vi "Catch_screw.vi"(7 "櫃子在哪?":enum16{"前面", "左邊", "右邊"}(ring), 8 "Error In":errorcluster) -> (0 "Error Out":errorcluster)   [LabVIEW 2019]
uses:
  WSCbot_V3_Toolkit.lvlibp/WSCBOTV3_Toolkit/IO/LowLevel/PulseCounter.ctl
  WSCbot_V3_Toolkit.lvlibp
panel:
  in  "螺桿高度":dbl(ring)=78.0 items=["物料櫃第一格"=0.0, "物料櫃第二格"=78.0, "螺帽夾取高度"=128.0, "螺帽瞄準"=250.0, "最高"=288.0]
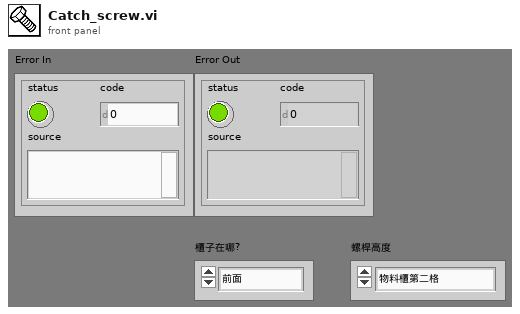
[diagram p1: front panel]
types:
  T1 = enum16{"Right_up", "Right_down", "Left_down", "Left_up", "left", "right", "up", "down"}
  T2 = typedef "WSCbot_V3_Toolkit.lvlibp/PulseCounter.ctl" = enum16{"CH1", "CH2", "CH3", "CH4", "CH5"}
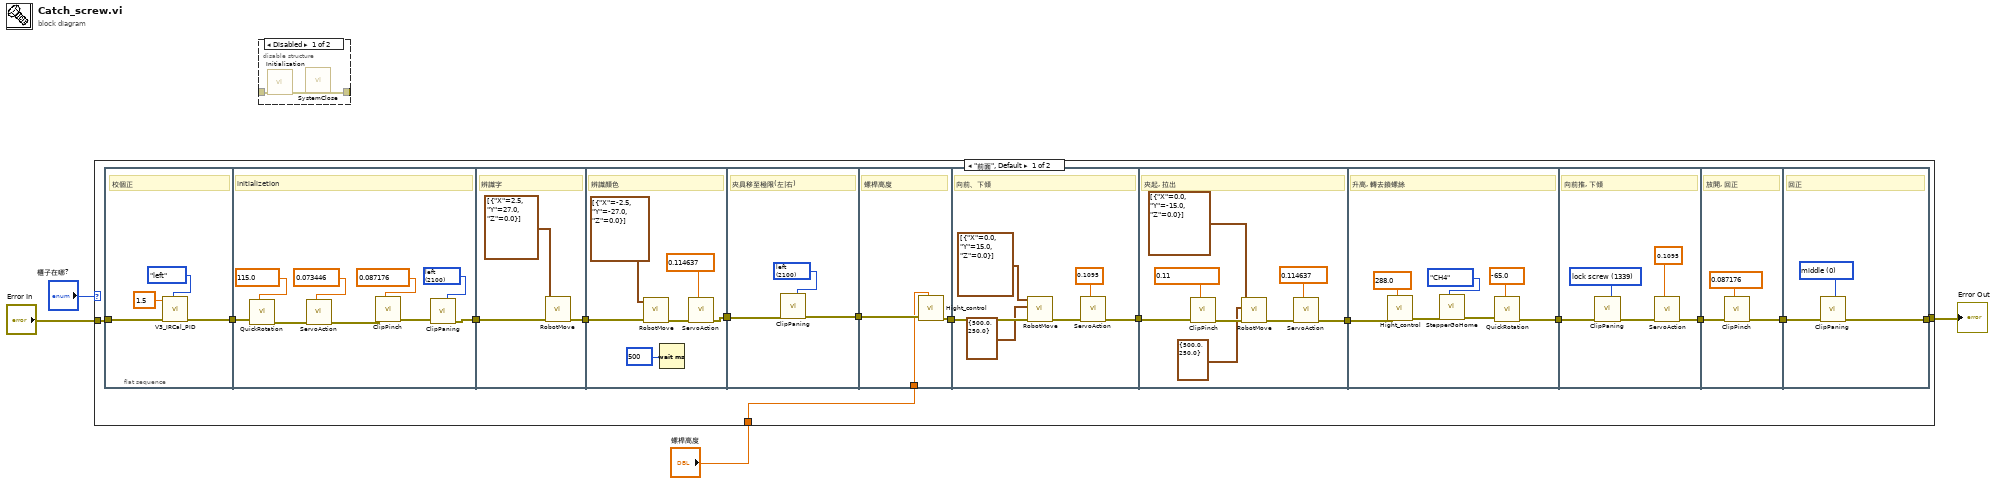
[diagram p0: block diagram]
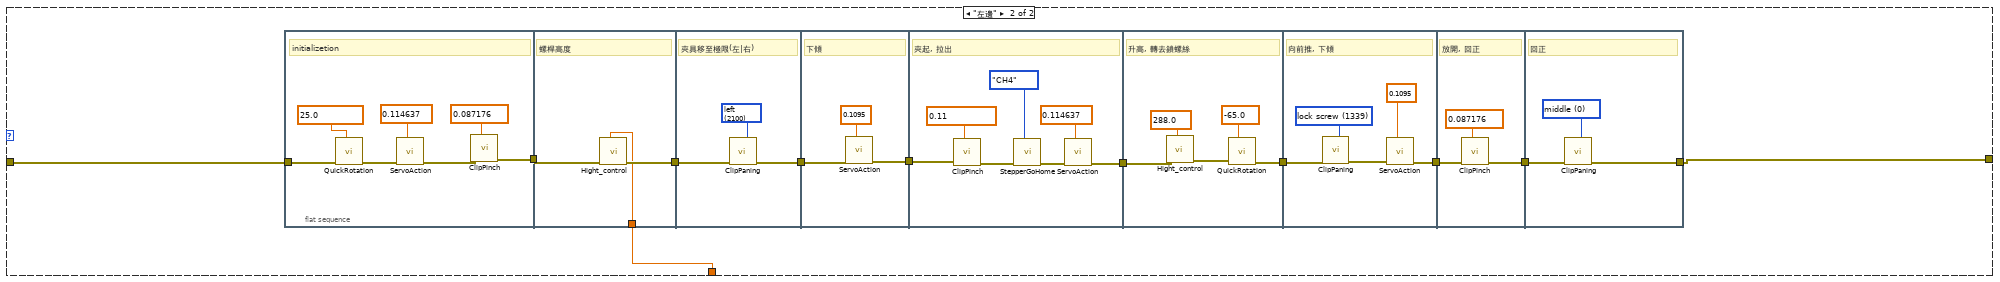
[diagram p2: hidden frame]
diagram:
  n1 = case shown="\"前面\", Default" "櫃子在哪?" {
    tunnel: [w10 w81] -> w4
    tunnel: "Error In" -> [w11 w80]
    tunnel: "螺桿高度" -> [w8 w79]
    frame "前面", Default {
      n2 = flat-sequence {
        tunnel: w11 -> [w21]
        tunnel: [w20] -> w5
        tunnel: [w24] -> w6
        tunnel: w5 -> [w26]
        tunnel: [w34] -> w7
        tunnel: w6 -> [w32]
        tunnel: [w37] -> w18
        tunnel: w7 -> [w40]
        tunnel: w18 -> [w42]
        tunnel: [w41] -> w9
        tunnel: [w45] -> w17
        tunnel: w9 -> [w46]
        tunnel: w8 -> [w44]
        tunnel: w17 -> [w50]
        tunnel: [w52] -> w16
        tunnel: [w58] -> w15
        tunnel: w16 -> [w59]
        tunnel: w15 -> [w65]
        tunnel: [w66] -> w14
        tunnel: w14 -> [w72]
        tunnel: [w68] -> w13
        tunnel: w13 -> [w75]
        tunnel: [w73] -> w12
        tunnel: w12 -> [w77]
        tunnel: [w76] -> w10
        frame #0 {
          # "校個正"
          n3 = call "V3_IRCal_PID.vi"("Direction"=T1."left", "Error In"=w21, "X_distance(V)"=1.5) -> ("Error Out"=w20:errorcluster)  [unwired: 7 in, 1 out]
        }
        frame #1 {
          w23 = 2100 items=["left"=2100, "right"=-3500, "lock screw"=1339, "middle"=0] ("location")
          w29 = 115.0 items=["Forward"=25.0, "Right"=115.0, "Left"=-65.0] ("螺桿面向")
          w28 = 0.087176 items=["pinch_up"=0.11, "release"=0.087176] ("pinch?")
          w27 = 0.073446 items=["up"=0.1095, "up_up"=0.114637, "down"=0.073446, "back"=0.037435, "back_back"=0.035] ("face_dir")
          # "initializetion"
          n4 = call "QuickRotation.vi"("螺桿面向"=w29, "Error In"=w26) -> ("Error Out"=w30:errorcluster)  [unwired: 9 in]
          n5 = call "ServoAction.vi"("face_dir"=w27, "Error In"=w30) -> ("Error Out"=w31:errorcluster)  [unwired: 9 in]
          n6 = call "ClipPinch.vi"("pinch?"=w28, "Error In"=w31) -> ("Error Out"=w25:errorcluster)  [unwired: 9 in]
          n7 = call "ClipPaning.vi"("Error In"=w25, "location"=w23) -> ("Error Out"=w24:errorcluster)  [unwired: 8 in]
        }
        frame #2 {
          # "辨識字"
          n8 = call "RobotMove.vi"("error in (no error)"=w32, "XYZ"=cluster{"X":dbl, "Y":dbl, "Z":dbl}[] [{"X"=2.5, "Y"=27.0, "Z"=0.0}]) -> ("error out"=w34:errorcluster)  [unwired: 9 in]
        }
        frame #3 {
          w36 = 0.114637 items=["up"=0.1095, "lock_up"=0.111528, "up_up"=0.114637, "down"=0.073446, "back"=0.037435, "back_back"=0.035] ("face_dir")
          # "辨識顏色"
          n9 = call "RobotMove.vi"("error in (no error)"=w40, "XYZ"=cluster{"X":dbl, "Y":dbl, "Z":dbl}[] [{"X"=-2.5, "Y"=-27.0, "Z"=0.0}]) -> ("error out"=w38:errorcluster)  [unwired: 9 in]
          n10 = Wait (ms)(milliseconds to wait=u32 500) -> ()  [unwired: 1 out]
          n11 = call "ServoAction.vi"("face_dir"=w36, "Error In"=w38) -> ("Error Out"=w37:errorcluster)  [unwired: 9 in]
        }
        frame #4 {
          w43 = 2100 items=["left"=2100, "right"=-3500, "lock screw"=1339, "middle"=0] ("location")
          # "夾具移至極限(左|右)"
          n12 = call "ClipPaning.vi"("Error In"=w42, "location"=w43) -> ("Error Out"=w41:errorcluster)  [unwired: 8 in]
        }
        frame #5 {
          # "螺桿高度"
          n13 = call "Hight_control.vi"("螺桿高度"=w44, "Error In"=w46) -> ("Error Out"=w45:errorcluster)  [unwired: 9 in]
        }
        frame #6 {
          w51 = 0.1095 items=["up"=0.1095, "up_up"=0.114637, "down"=0.073446, "back"=0.037435, "back_back"=0.035] ("face_dir")
          # "向前、下傾"
          n14 = call "RobotMove.vi"("error in (no error)"=w50, "Speed/ACC"=cluster{dbl, dbl} {500.0, 250.0}, "XYZ"=cluster{"X":dbl, "Y":dbl, "Z":dbl}[] [{"X"=0.0, "Y"=15.0, "Z"=0.0}]) -> ("error out"=w49:errorcluster)  [unwired: 8 in]
          n15 = call "ServoAction.vi"("face_dir"=w51, "Error In"=w49) -> ("Error Out"=w52:errorcluster)  [unwired: 9 in]
        }
        frame #7 {
          w57 = 0.114637 items=["up"=0.1095, "up_up"=0.114637, "down"=0.073446, "back"=0.037435, "back_back"=0.035] ("face_dir")
          w60 = 0.11 items=["pinch_up"=0.11, "release"=0.087176] ("pinch?")
          # "夾起, 拉出"
          n16 = call "ClipPinch.vi"("pinch?"=w60, "Error In"=w59) -> ("Error Out"=w56:errorcluster)  [unwired: 9 in]
          n17 = call "RobotMove.vi"("error in (no error)"=w56, "Speed/ACC"=cluster{dbl, dbl} {500.0, 250.0}, "XYZ"=cluster{"X":dbl, "Y":dbl, "Z":dbl}[] [{"X"=0.0, "Y"=-15.0, "Z"=0.0}]) -> ("error out"=w55:errorcluster)  [unwired: 8 in]
          n18 = call "ServoAction.vi"("face_dir"=w57, "Error In"=w55) -> ("Error Out"=w58:errorcluster)  [unwired: 9 in]
        }
        frame #8 {
          w64 = 288.0 items=["物料櫃第一格"=0.0, "物料櫃第二格"=78.0, "螺帽夾取高度"=128.0, "螺帽瞄準"=250.0, "最高"=288.0] ("螺桿高度")
          w67 = -65.0 items=["Forward"=25.0, "Right"=115.0, "Left"=-65.0] ("螺桿面向")
          # "升高, 轉去鎖螺絲"
          n19 = call "Hight_control.vi"("螺桿高度"=w64, "Error In"=w65) -> ("Error Out"=w62:errorcluster)  [unwired: 9 in]
          n20 = call "StepperGoHome.vi"("PulseCounterChanel"=PulseCounter."CH4", "Error In"=w62) -> ("Error Out"=w61:errorcluster)  [unwired: 7 in, 2 out]
          n21 = call "QuickRotation.vi"("螺桿面向"=w67, "Error In"=w61) -> ("Error Out"=w66:errorcluster)  [unwired: 9 in]
        }
        frame #9 {
          w69 = 0.1095 items=["up"=0.1095, "up_up"=0.114637, "down"=0.073446, "back"=0.037435, "back_back"=0.035] ("face_dir")
          w71 = 1339 items=["left"=2100, "right"=-3500, "lock screw"=1339, "middle"=0] ("location")
          # "向前推, 下傾"
          n22 = call "ClipPaning.vi"("Error In"=w72, "location"=w71) -> ("Error Out"=w70:errorcluster)  [unwired: 8 in]
          n23 = call "ServoAction.vi"("face_dir"=w69, "Error In"=w70) -> ("Error Out"=w68:errorcluster)  [unwired: 9 in]
        }
        frame #10 {
          w74 = 0.087176 items=["pinch_up"=0.11, "release"=0.087176] ("pinch?")
          # "放開, 回正"
          n24 = call "ClipPinch.vi"("pinch?"=w74, "Error In"=w75) -> ("Error Out"=w73:errorcluster)  [unwired: 9 in]
        }
        frame #11 {
          w78 = 0 items=["left"=2100, "right"=-3500, "lock screw"=1339, "middle"=0] ("location")
          # "回正"
          n25 = call "ClipPaning.vi"("Error In"=w77, "location"=w78) -> ("Error Out"=w76:errorcluster)  [unwired: 8 in]
        }
      }
    }
    frame "左邊" {
      n26 = flat-sequence {
        tunnel: [w93] -> w89
        tunnel: w80 -> [w91]
        tunnel: w89 -> [w99]
        tunnel: [w98] -> w88
        tunnel: w79 -> [w97]
        tunnel: [w102] -> w87
        tunnel: w88 -> [w100]
        tunnel: w87 -> [w104]
        tunnel: [w105] -> w86
        tunnel: [w107] -> w85
        tunnel: w86 -> [w109]
        tunnel: w85 -> [w115]
        tunnel: [w116] -> w84
        tunnel: w84 -> [w122]
        tunnel: [w118] -> w83
        tunnel: w83 -> [w125]
        tunnel: [w123] -> w82
        tunnel: w82 -> [w127]
        tunnel: [w126] -> w81
        frame #0 {
          w90 = 25.0 items=["Forward"=25.0, "Right"=115.0, "Left"=-65.0] ("螺桿面向")
          w95 = 0.087176 items=["pinch_up"=0.11, "release"=0.087176] ("pinch?")
          w96 = 0.114637 items=["up"=0.1095, "up_up"=0.114637, "down"=0.073446, "back"=0.037435, "back_back"=0.035] ("face_dir")
          # "initializetion"
          n27 = call "QuickRotation.vi"("螺桿面向"=w90, "Error In"=w91) -> ("Error Out"=w92:errorcluster)  [unwired: 9 in]
          n28 = call "ServoAction.vi"("face_dir"=w96, "Error In"=w92) -> ("Error Out"=w94:errorcluster)  [unwired: 9 in]
          n29 = call "ClipPinch.vi"("pinch?"=w95, "Error In"=w94) -> ("Error Out"=w93:errorcluster)  [unwired: 9 in]
        }
        frame #1 {
          # "螺桿高度"
          n30 = call "Hight_control.vi"("螺桿高度"=w97, "Error In"=w99) -> ("Error Out"=w98:errorcluster)  [unwired: 9 in]
        }
        frame #2 {
          w101 = 2100 items=["left"=2100, "right"=-3500, "lock screw"=1339, "middle"=0] ("location")
          # "夾具移至極限(左|右)"
          n31 = call "ClipPaning.vi"("Error In"=w100, "location"=w101) -> ("Error Out"=w102:errorcluster)  [unwired: 8 in]
        }
        frame #3 {
          w103 = 0.1095 items=["up"=0.1095, "up_up"=0.114637, "down"=0.073446, "back"=0.037435, "back_back"=0.035] ("face_dir")
          # "下傾"
          n32 = call "ServoAction.vi"("face_dir"=w103, "Error In"=w104) -> ("Error Out"=w105:errorcluster)  [unwired: 9 in]
        }
        frame #4 {
          w106 = 0.114637 items=["up"=0.1095, "up_up"=0.114637, "down"=0.073446, "back"=0.037435, "back_back"=0.035] ("face_dir")
          w112 = 0.11 items=["pinch_up"=0.11, "release"=0.087176] ("pinch?")
          # "夾起, 拉出"
          n33 = call "ClipPinch.vi"("pinch?"=w112, "Error In"=w109) -> ("Error Out"=w111:errorcluster)  [unwired: 9 in]
          n34 = call "StepperGoHome.vi"("PulseCounterChanel"=PulseCounter."CH4", "Error In"=w111) -> ("Error Out"=w108:errorcluster)  [unwired: 7 in, 2 out]
          n35 = call "ServoAction.vi"("face_dir"=w106, "Error In"=w108) -> ("Error Out"=w107:errorcluster)  [unwired: 9 in]
        }
        frame #5 {
          w113 = 288.0 items=["物料櫃第一格"=0.0, "物料櫃第二格"=78.0, "螺帽夾取高度"=128.0, "螺帽瞄準"=250.0, "最高"=288.0] ("螺桿高度")
          w117 = -65.0 items=["Forward"=25.0, "Right"=115.0, "Left"=-65.0] ("螺桿面向")
          # "升高, 轉去鎖螺絲"
          n36 = call "Hight_control.vi"("螺桿高度"=w113, "Error In"=w115) -> ("Error Out"=w114:errorcluster)  [unwired: 9 in]
          n37 = call "QuickRotation.vi"("螺桿面向"=w117, "Error In"=w114) -> ("Error Out"=w116:errorcluster)  [unwired: 9 in]
        }
        frame #6 {
          w119 = 0.1095 items=["up"=0.1095, "up_up"=0.114637, "down"=0.073446, "back"=0.037435, "back_back"=0.035] ("face_dir")
          w121 = 1339 items=["left"=2100, "right"=-3500, "lock screw"=1339, "middle"=0] ("location")
          # "向前推, 下傾"
          n38 = call "ClipPaning.vi"("Error In"=w122, "location"=w121) -> ("Error Out"=w120:errorcluster)  [unwired: 8 in]
          n39 = call "ServoAction.vi"("face_dir"=w119, "Error In"=w120) -> ("Error Out"=w118:errorcluster)  [unwired: 9 in]
        }
        frame #7 {
          w124 = 0.087176 items=["pinch_up"=0.11, "release"=0.087176] ("pinch?")
          # "放開, 回正"
          n40 = call "ClipPinch.vi"("pinch?"=w124, "Error In"=w125) -> ("Error Out"=w123:errorcluster)  [unwired: 9 in]
        }
        frame #8 {
          w128 = 0 items=["left"=2100, "right"=-3500, "lock screw"=1339, "middle"=0] ("location")
          # "回正"
          n41 = call "ClipPaning.vi"("Error In"=w127, "location"=w128) -> ("Error Out"=w126:errorcluster)  [unwired: 8 in]
        }
      }
    }
  }
  "Error Out" <- w4
  n42 = disable-structure shown="Disabled" {
    disable-tunnel: [w130 _] -> _
    disable-tunnel: _ -> [w129 _]
    frame Disabled {
      n43 = call "Initialization.vi"("Error In"=w129) -> ("Error Out"=w130:errorcluster)  [unwired: 10 in]
      n44 = call "SystemClose.vi"() -> ()  [unwired: 3 in, 1 out]
    }
    frame Enabled {
    }
  }
